vi "EVM_Sweep_Only_R_S_2.vi"() -> ()   [LabVIEW 2023, in "EVM.lvlib"]
uses:
  lib/CTL/LitePoint_EVM_SG.ctl
  lib/CTL/LitePoint_EVM_SA.ctl
  EVM.lvlib
  lib/LitePoints/LitePoints.lvlib
  lib/FTDI/JIO/CLC_JIO_FTDI.lvlib
  lib/R_S/R_S.lvlib
panel:
  in  "SGpower":i32=-10
  in  "BFIC_ele_stop":i32=15
  in  "BFIC_ele_res":i32=15
  in  "BFIC_ele_start":i32
  in  "BFIC_com_stop":i32=15
  in  "BFIC_com_res":i32=15
  in  "BFIC_com_start":i32
  in  "UD_att_stop":i32=255
  in  "UD_att_res":i32=255
  in  "UD_att_start":i32
  out "UD_att":i32=255
  out "BFIC_com_step":i32=15
  out "BFIC_ele_step":i32=15
  in  "TRXmode":u16(ring)=1 items=["Tx"=1, "Rx"=2]
  in  "Polarity":u16(ring) items=["H", "V"]
  out "floder Exist?":bool=TRUE
  in  "Waiting \nTime(ms)":u32=1
  in  "FileNote":string="test16_wayne_MCS11"
  in  "SG":refnum<visa-resource-name>="TCPIP::192.168.88.12::hislip0::INSTR"
  in  "SA":refnum<visa-resource-name>="TCPIP0::LAB_XBeam-NB::inst0::INSTR"
  out "Spectrum Data":cluster{"X":dbl, "Y":dbl}[](graph)
  # "TMYTEK_CLC_JIO_R&S_EVM"
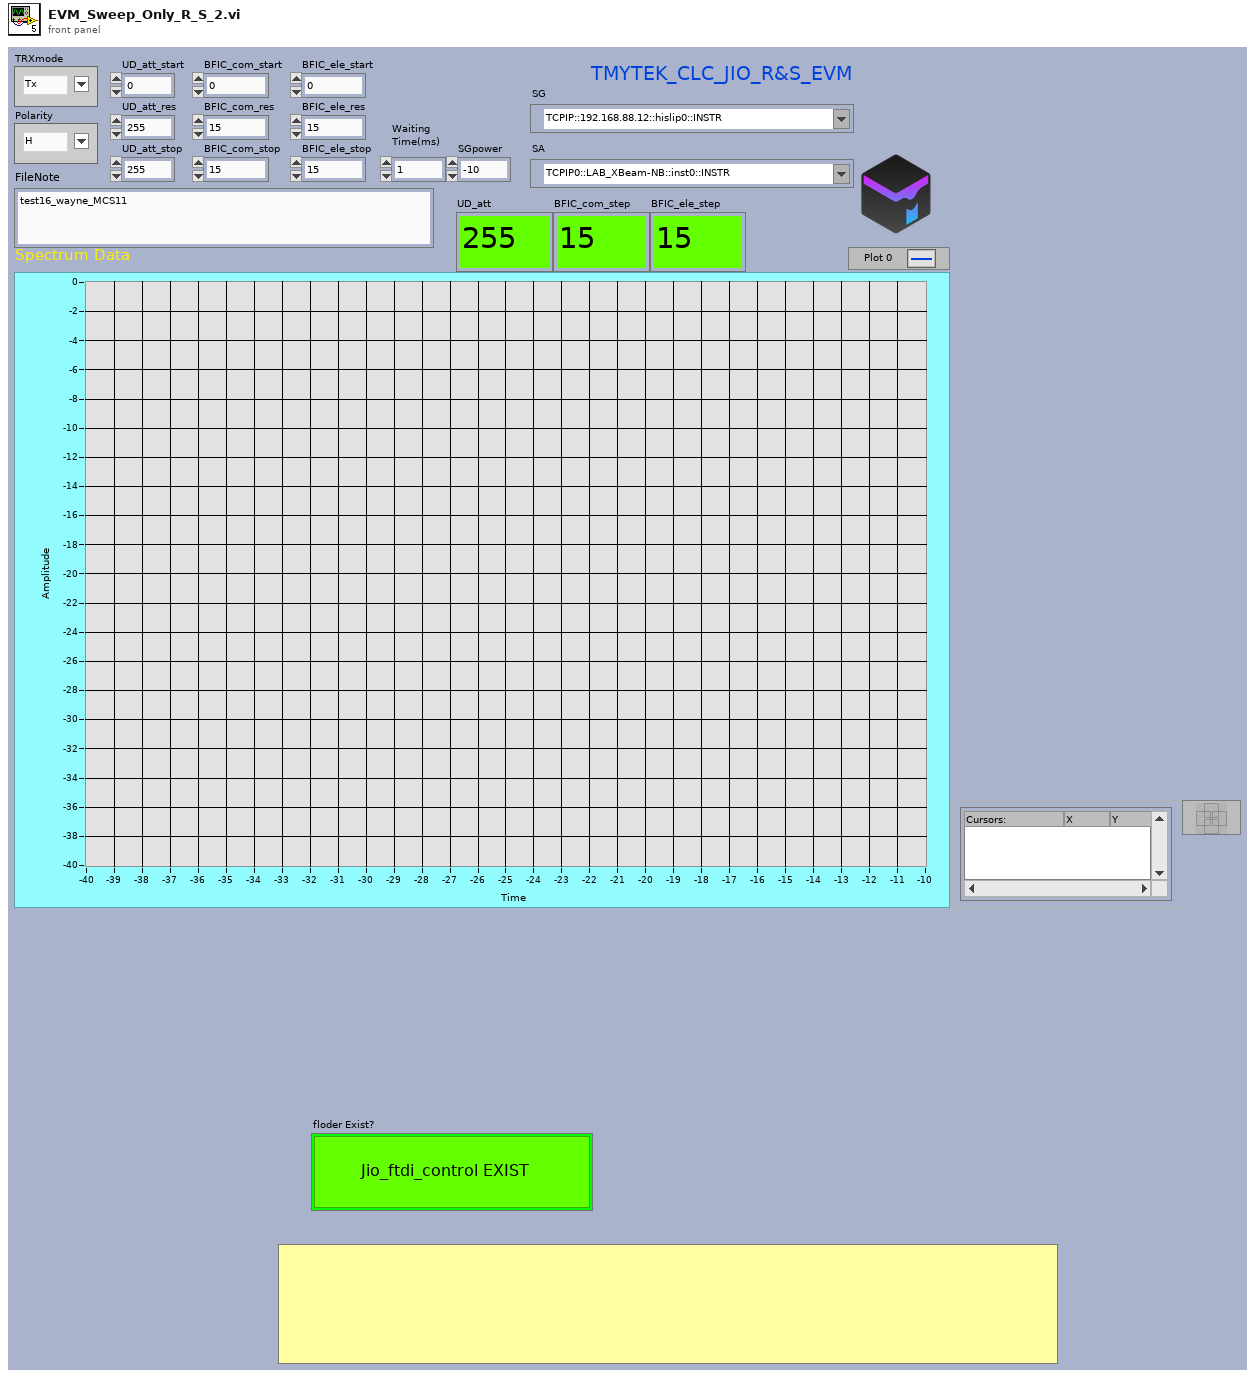
[diagram p1: front panel]
types:
  T1 = typedef "LitePoint_EVM_SG.ctl" = enum16{"Init", "Close", "set_SG", "AdjustLevel", "byPass", "RF_ON", "RF_OFF"}
  T2 = typedef "LitePoint_EVM_SA.ctl" = enum16{"Init", "Close", "set_SA", "get_EVM", "byPass", "getPower"}
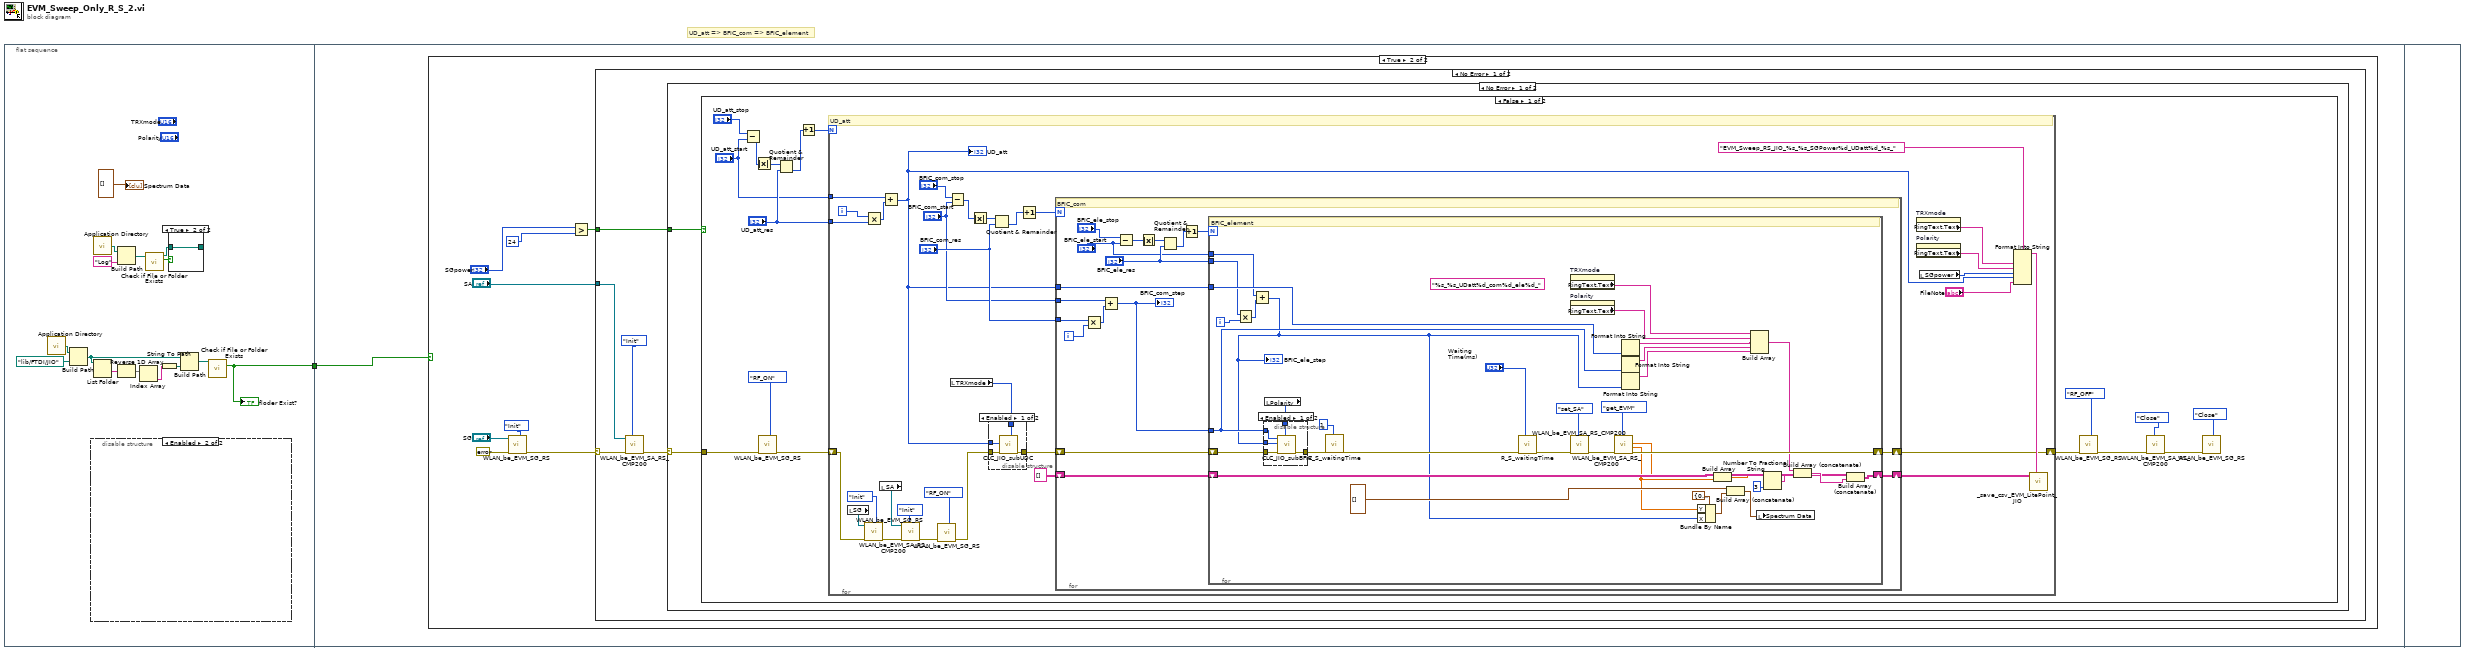
[diagram p0: block diagram]
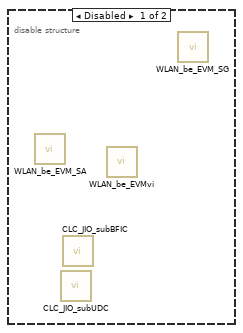
[diagram p2: hidden frame]
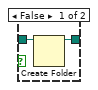
[diagram p3: hidden frame]
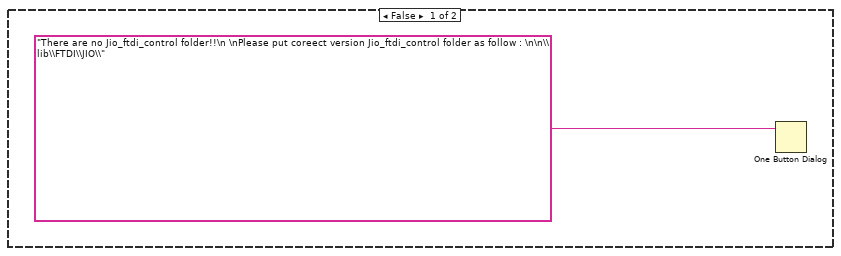
[diagram p4: hidden frame]
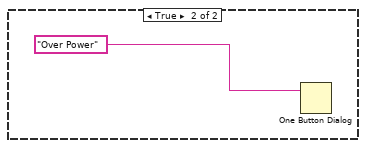
[diagram p7: hidden frame]
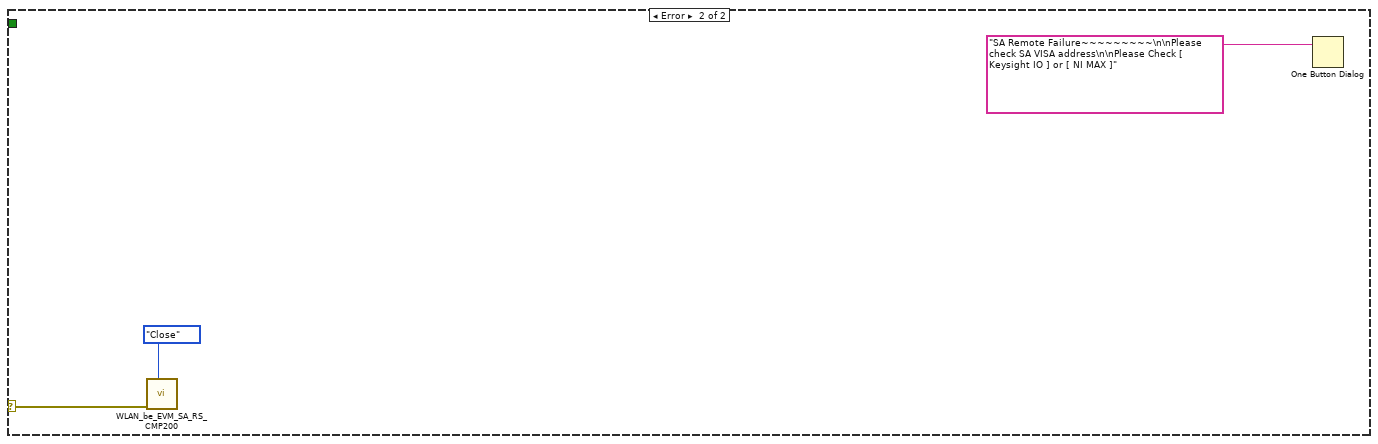
[diagram p8: hidden frame]
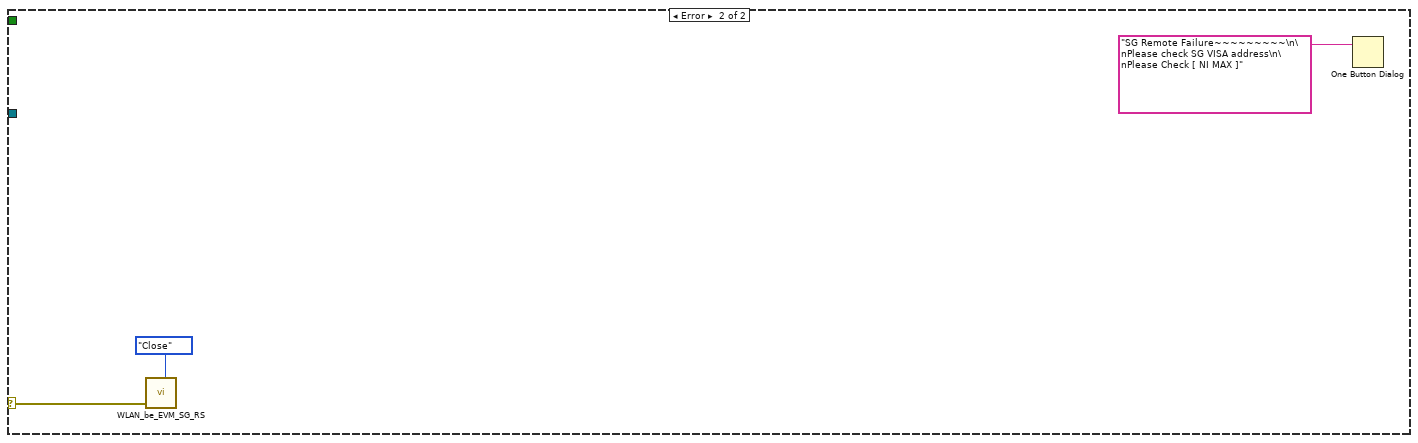
[diagram p9: hidden frame]
diagram:
  # "UD_att => BFIC_com => BFIC_element"
  n1 = flat-sequence {
    tunnel: [w2] -> w1
    tunnel: w1 -> [w20]
    frame #0 {
      n2 = call <vilib>:"Application Directory.vi"() -> ("Application Directory"=w8:path)
      n3 = Build Path(base path=w8, name or relative path=path "lib/FTDI/JIO") -> (appended path=w9:path)
      n4 = disable-structure shown="Enabled" {
        frame Disabled {
          n5 = call "WLAN_be_EVM_SA.vi"() -> ()  [unwired: 8 in, 4 out]
          n6 = call "CLC_JIO_subUDC.vi"() -> ()  [unwired: 10 in, 2 out]
          n7 = call "CLC_JIO_subBFIC.vi"() -> ()  [unwired: 10 in, 2 out]
          n8 = call "WLAN_be_EVMvi.vi"() -> ()  [unwired: 8 in, 4 out]
          n9 = call "WLAN_be_EVM_SG.vi"() -> ()  [unwired: 10 in, 2 out]
        }
        frame Enabled {
        }
      }
      n10 = call <vilib>:"Application Directory.vi"() -> ("Application Directory"=w15:path)
      n11 = List Folder(path=w9) -> (folder names=w4:string[])  [unwired: 3 in, 3 out]
      n12 = Reverse 1D Array(array=w4) -> (reversed array=w5:string[])
      n13 = Build Path(base path=w15, name or relative path="Log") -> (appended path=w12:path)
      n14 = Index Array(array=w5) -> (element=w6:string)  [unwired: 1 in]
      n15 = call <vilib>:"Check if File or Folder Exists.vi"("path"=w12) -> ("file or folder exists?"=w14:bool, "dup path"=w13:path)  [unwired: 8 in, 1 out]
      n16 = String To Path(string=w6) -> (path=w7:path)
      n17 = case shown="True" w14 {
        tunnel: w13 -> [w18 w19]
        tunnel: [w17 w19] -> _
        frame False {
          n18 = Create Folder(path (use dialog)=w18) -> (created path=w17:path)  [unwired: 2 in, 2 out]
        }
        frame True {
        }
      }
      n19 = Build Path(base path=w9, name or relative path=w7) -> (appended path=w10:path)
      n20 = call <vilib>:"Check if File or Folder Exists.vi"("path"=w10) -> ("file or folder exists?"=w2:bool)  [unwired: 8 in, 2 out]
      "floder Exist?" <- w2
      "Spectrum Data" <- cluster{"X":dbl, "Y":dbl}[] [] ("XY Graph")
    }
    frame #1 {
      n21 = case shown="True" w20 {
        frame False {
          n22 = One Button Dialog(message="There are no Jio_ftdi_control folder!!\n \nPlease put coreect version Jio_ftdi_control folder as follow : \n\n\\lib\\FTDI\\JIO\\") -> ()  [unwired: 1 in, 1 out]
        }
        frame True {
          n23 = call "WLAN_be_EVM_SG_RS.vi"("Function_SG"=LitePoint_EVM_SG."Init", "error in"=errorcluster {"status"=FALSE, "code"=0, "source"=""} ("error in (no error)"), "VISA IN"="SG") -> ("error out"=w24:errorcluster)  [unwired: 7 in, 1 out]
          n24 = Greater?(x="SGpower", y=24) -> (0:w28:bool)
          n25 = case shown="No Error" w24 {
            selector: w24 -> [w33 w154]
            tunnel: "SA" -> [w31 _]
            tunnel: w28 -> [w34 _]
            frame No Error {
              n26 = call "WLAN_be_EVM_SA_RS_CMP200.vi"("Function"=LitePoint_EVM_SA."Init", "error in"=w33, "VISA IN"=w31) -> ("error out"=w32:errorcluster)  [unwired: 5 in, 3 out]
              n27 = case shown="No Error" w32 {
                selector: w32 -> [w35 w151]
                tunnel: w34 -> [w36 _]
                frame No Error {
                  n28 = case shown="False" w36 {
                    tunnel: w35 -> [w52 _]
                    frame False {
                      n29 = Subtract(x="UD_att_stop", y="UD_att_start") -> (x-y=w44:i32)
                      n30 = Absolute Value(x=w44) -> (abs(x)=w41:i32)
                      n31 = call "WLAN_be_EVM_SG_RS.vi"("Function_SG"=LitePoint_EVM_SG."RF_ON", "error in"=w52) -> ("error out"=w50:errorcluster)  [unwired: 8 in, 1 out]
                      n32 = Quotient & Remainder(x=w41, y="UD_att_res") -> (floor(x/y)=w42:i32)  [unwired: 1 out]
                      n33 = Increment(x=w42) -> (x+1=w38:i32)
                      n34 = for {
                        N: w38 -> [_]
                        shift-right: [w76] -> w49
                        shift-left: w50 -> [w63]
                        tunnel: "UD_att_res" -> [w73]
                        tunnel: "UD_att_start" -> [w72]
                        i -> [w75]
                        # "UD_att"
                        n35 = local read "SG"() -> (w60:refnum<visa-resource-name>)
                        n36 = call "WLAN_be_EVM_SG_RS.vi"("Function_SG"=LitePoint_EVM_SG."Init", "error in"=w63, "VISA IN"=w60) -> ("error out"=w61:errorcluster)  [unwired: 7 in, 1 out]
                        n37 = Multiply(x=w75, y=w73) -> (x*y=w74:i32)
                        n38 = local read "SA"() -> (w59:refnum<visa-resource-name>)
                        n39 = Add(x=w72, y=w74) -> (x+y=w54:i32)
                        "UD_att" <- w54
                        n40 = call "WLAN_be_EVM_SA_RS_CMP200.vi"("Function"=LitePoint_EVM_SA."Init", "error in"=w61, "VISA IN"=w59) -> ("error out"=w57:errorcluster)  [unwired: 5 in, 3 out]
                        n41 = call "WLAN_be_EVM_SG_RS.vi"("Function_SG"=LitePoint_EVM_SG."RF_ON", "error in"=w57) -> ("error out"=w56:errorcluster)  [unwired: 8 in, 1 out]
                        n42 = Subtract(x="BFIC_com_stop", y="BFIC_com_start") -> (x-y=w71:i32)
                        n43 = local read "TRXmode"() -> (w82:u16)
                        n44 = Absolute Value(x=w71) -> (abs(x)=w70:i32)
                        n45 = disable-structure shown="Enabled" {
                          disable-tunnel: [w88 w89] -> w84
                          disable-tunnel: w56 -> [w87 w89]
                          disable-tunnel: w82 -> [w86 _]
                          disable-tunnel: w54 -> [w85 _]
                          frame Enabled {
                            n46 = call "CLC_JIO_subUDC.vi"("Mode"=w86, "error in"=w87, "ud att"=w85) -> ("error out"=w88:errorcluster)  [unwired: 7 in, 1 out]
                          }
                          frame Disabled {
                          }
                        }
                        n47 = Quotient & Remainder(x=w70, y="BFIC_com_res") -> (floor(x/y)=w66:i32)  [unwired: 1 out]
                        n48 = Increment(x=w66) -> (x+1=w65:i32)
                        n49 = for {
                          N: w65 -> [_]
                          shift-right: [w104] -> w83
                          shift-left: string[][] [] -> [w105]
                          tunnel: w54 -> [w103]
                          shift-right: [w102] -> w76
                          shift-left: w84 -> [w106]
                          tunnel: "BFIC_com_res" -> [w98]
                          tunnel: "BFIC_com_start" -> [w97]
                          i -> [w100]
                          # "BFIC_com"
                          n50 = Multiply(x=w98, y=w100) -> (x*y=w101:i32)
                          n51 = Add(x=w97, y=w101) -> (x+y=w99:i32)
                          "BFIC_com_step" <- w99
                          n52 = Subtract(x="BFIC_ele_stop", y="BFIC_ele_start") -> (x-y=w95:i32)
                          n53 = Absolute Value(x=w95) -> (abs(x)=w96:i32)
                          n54 = Quotient & Remainder(x=w96, y="BFIC_ele_res") -> (floor(x/y)=w93:i32)  [unwired: 1 out]
                          n55 = Increment(x=w93) -> (x+1=w90:i32)
                          n56 = for {
                            N: w90 -> [_]
                            shift-right: [w140] -> w104
                            shift-left: w105 -> [w139]
                            tunnel: w99 -> [w134]
                            tunnel: w103 -> [w135]
                            shift-right: [w132] -> w102
                            shift-left: w106 -> [w138]
                            tunnel: "BFIC_ele_res" -> [w129]
                            tunnel: "BFIC_ele_start" -> [w128]
                            i -> [w130]
                            (unwired) "%s_%s_UDatt%d_com%d_ele%d_" ("format string")
                            # "BFIC_element"
                            n57 = Multiply(x=w129, y=w130) -> (x*y=w131:i32)
                            n58 = Add(x=w128, y=w131) -> (x+y=w107:i32)
                            "BFIC_ele_step" <- w107
                            n59 = local read "Polarity"() -> (w133:u16)
                            n60 = disable-structure shown="Enabled" {
                              disable-tunnel: w138 -> [w147 w148]
                              disable-tunnel: [w146 w148] -> w137
                              disable-tunnel: w107 -> [w145 _]
                              disable-tunnel: w134 -> [w144 _]
                              disable-tunnel: w133 -> [w143 _]
                              frame Enabled {
                                n61 = call "CLC_JIO_subBFIC.vi"("pol"=w143, "error in"=w147, "ele"=w145, "com"=w144) -> ("error out"=w146:errorcluster)  [unwired: 6 in, 1 out]
                              }
                              frame Disabled {
                              }
                            }
                            n62 = call "R_S_waitingTime.vi"("Waiting Time(ms)"=u32 1, "error in"=w137) -> ("error out"=w108:errorcluster)  [unwired: 9 in]
                            n63 = call "R_S_waitingTime.vi"("Waiting Time(ms)"="Waiting \nTime(ms)", "error in"=w108) -> ("error out"=w121:errorcluster)  [unwired: 9 in]
                            n64 = property on="TRXmode" class="Ring (strict)"() -> ("RingText.Text"=w116:string)  [unwired: 2 in, 2 out]
                            n65 = property on="Polarity" class="Ring (strict)"() -> ("RingText.Text"=w115:string)  [unwired: 2 in, 2 out]
                            n66 = call "WLAN_be_EVM_SA_RS_CMP200.vi"("Function"=LitePoint_EVM_SA."set_SA", "error in"=w121) -> ("error out"=w110:errorcluster)  [unwired: 6 in, 3 out]
                            n67 = call "WLAN_be_EVM_SA_RS_CMP200.vi"("Function"=LitePoint_EVM_SA."get_EVM", "error in"=w110) -> ("error out"=w132:errorcluster, "EVM"=w122:dbl, "Power"=w109:dbl)  [unwired: 6 in, 1 out]
                            n68 = Format Into String(w135) -> (resulting string=w114:string)  [unwired: 3 in, 1 out]
                            n69 = Format Into String(w134) -> (resulting string=w113:string)  [unwired: 3 in, 1 out]
                            n70 = Format Into String(w107) -> (resulting string=w112:string)  [unwired: 3 in, 1 out]
                            n71 = Bundle By Name(cluster=cluster{"X":dbl, "Y":dbl} {"X"=0.0, "Y"=0.0} ("element"), "Y"=w122, "X"=w107) -> (w126:cluster{"X":dbl, "Y":dbl})
                            n72 = Build Array(w109, w122) -> (w118:dbl[])
                            n73 = Build Array (concatenate)(cluster{"X":dbl, "Y":dbl}[] [] ("XY Graph"), w126) -> (w125:cluster{"X":dbl, "Y":dbl}[])
                            n74 = Build Array(w116, w115, w114, w113, w112) -> (w111:string[])
                            n75 = local write "Spectrum Data"(w125) -> ()
                            n76 = Number To Fractional String(number=w118, precision (6)=i16 3) -> (F-format string=w117:string[])  [unwired: 2 in]
                            n77 = Build Array (concatenate)(w111, w117) -> (w141:string[])
                            n78 = Build Array (concatenate)(w139, w141) -> (w140:string[][])
                          }
                        }
                        n79 = property on="TRXmode" class="Ring (strict)"() -> ("RingText.Text"=w78:string)  [unwired: 2 in, 2 out]
                        n80 = property on="Polarity" class="Ring (strict)"() -> ("RingText.Text"=w79:string)  [unwired: 2 in, 2 out]
                        n81 = local read "SGpower"() -> (w53:i32)
                        n82 = Format Into String(format string="EVM_Sweep_RS_JIO_%s_%s_SGPower%d_UDatt%d_%s_" ("delimiter (\\t)"), w78, w79, w53, w54, "FileNote") -> (resulting string=w80:string)  [unwired: 2 in, 1 out]
                        n83 = call "_save_csv_EVM_LitePoint_JIO.vi"("delimiter (\\t)"=w80, "array in"=w83) -> ()  [unwired: 9 in, 1 out]
                      }
                      n84 = call "WLAN_be_EVM_SG_RS.vi"("Function_SG"=LitePoint_EVM_SG."RF_OFF", "error in"=w49) -> ("error out"=w46:errorcluster)  [unwired: 8 in, 1 out]
                      n85 = call "WLAN_be_EVM_SA_RS_CMP200.vi"("Function"=LitePoint_EVM_SA."Close", "error in"=w46) -> ("error out"=w45:errorcluster)  [unwired: 6 in, 3 out]
                      n86 = call "WLAN_be_EVM_SG_RS.vi"("Function_SG"=LitePoint_EVM_SG."Close", "error in"=w45) -> ()  [unwired: 8 in, 2 out]
                    }
                    frame True {
                      n87 = One Button Dialog(message="Over Power") -> ()  [unwired: 1 in, 1 out]
                    }
                  }
                }
                frame Error {
                  n88 = call "WLAN_be_EVM_SA_RS_CMP200.vi"("Function"=LitePoint_EVM_SA."Close", "error in"=w151) -> ()  [unwired: 6 in, 4 out]
                  n89 = One Button Dialog(message="SA Remote Failure~~~~~~~~~\n\nPlease check SA VISA address\n\nPlease Check [ Keysight IO ] or [ NI MAX ]") -> ()  [unwired: 1 in, 1 out]
                }
              }
            }
            frame Error {
              n90 = call "WLAN_be_EVM_SG_RS.vi"("Function_SG"=LitePoint_EVM_SG."Close", "error in"=w154) -> ()  [unwired: 8 in, 2 out]
              n91 = One Button Dialog(message="SG Remote Failure~~~~~~~~~\n\nPlease check SG VISA address\n\nPlease Check [ NI MAX ]") -> ()  [unwired: 1 in, 1 out]
            }
          }
        }
      }
    }
    frame #2 {
    }
  }
